vi "IKHinterface - initialize.vi"(8 "error in (no error)":errorcluster, 11 "EARTHLib.IKHInterface":refnum<k7>) -> (0 "error out":errorcluster, 3 "EARTHLib.IKHInterface 2":refnum<k7>)   [LabVIEW 2015]
panel:
  out "IsInitialized":i32
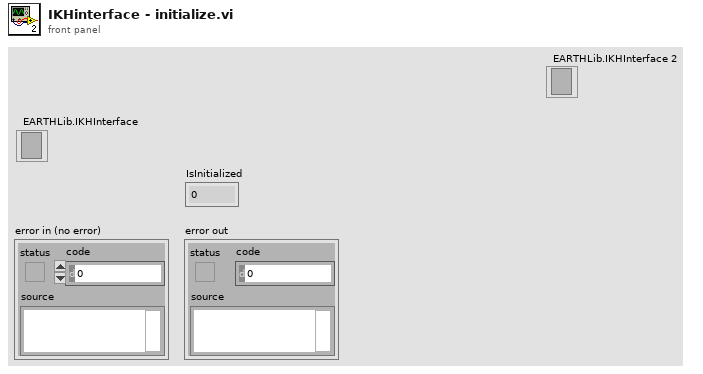
[diagram p1: front panel]
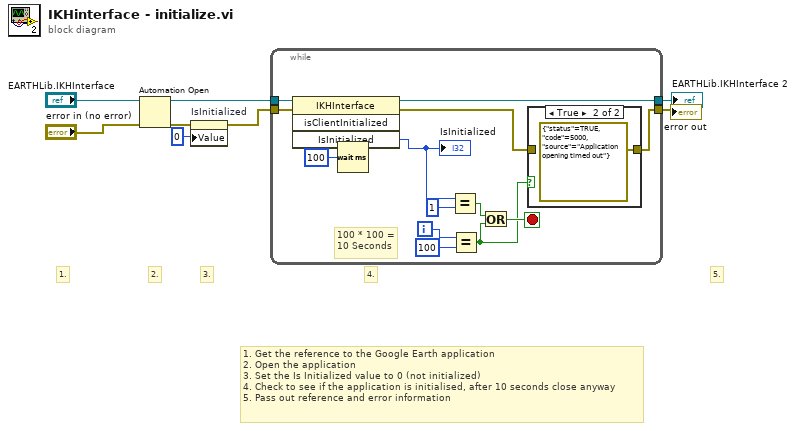
[diagram p0: block diagram]
diagram:
  # "1. Get the reference to the Google Earth application\n2. Open the application\n3. Set the Is Initialized value to 0 (not initialized)\n4. Check to see if the application is initialised, after 10 seconds close anyway\n5. Pass out reference and error information"
  # "5."
  # "4."
  # "3."
  # "2."
  # "1."
  n1 = Automation Open(error in (no error)="error in (no error)", Automation Refnum="EARTHLib.IKHInterface") -> (Automation Refnum=w7:refnum<k7>, error out=w6:errorcluster)  [unwired: 2 in]
  n2 = property on="IsInitialized" class="DigNum (strict)"(error in=w6, "Value"=0 ("IsInitialized")) -> (error out=w5:errorcluster)  [unwired: 1 in, 1 out]
  n3 = while {
    tunnel: [w10] -> w2
    tunnel: [w21] -> w1
    tunnel: w7 -> [w20]
    tunnel: w5 -> [w19]
    i -> [w14]
    stop <- w15 stop-if-true
    # "100 * 100 =\n10 Seconds"
    n4 = invoke class="IKHInterface" method="isClientInitialized"(reference=w20, error in=w19) -> (reference out=w21:refnum<k7>, error out=w11:errorcluster, "IsInitialized"=w9:i32)  [unwired: 2 in, 1 out]
    "IsInitialized" <- w9
    n5 = Wait (ms)(milliseconds to wait=u32 100) -> ()  [unwired: 1 out]
    n6 = Equal?(x=w9, y=1) -> (x = y?=w16:bool)
    n7 = Equal?(x=w14, y=100) -> (x = y?=w12:bool)
    n8 = Or(x=w16, y=w12) -> (x .or. y?=w15:bool)
    n9 = case shown="True" w12 {
      tunnel: w11 -> [w22 _]
      tunnel: [w22 errorcluster {"status"=TRUE, "code"=5000, "source"="Application opening timed out"} ("error out")] -> w10
      frame False {
      }
      frame True {
      }
    }
  }
  "error out" <- w2
  "EARTHLib.IKHInterface 2" <- w1
